vi "OpenLandscape.vi"() -> (1 "Landscape":string[][](array[string]), 2 "Slides":path)   [LabVIEW 2010]
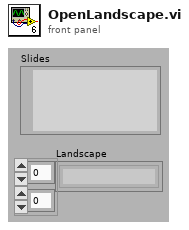
[diagram p1: front panel]
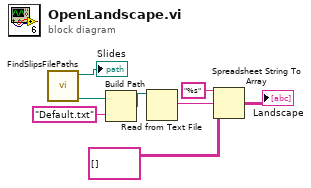
[diagram p0: block diagram]
diagram:
  n1 = call "FindSlipsFilePaths.vi"() -> ("Playlists"=w1:path, "Slides"=→"Slides":path)  [unwired: 2 in, 3 out]
  n2 = Build Path(base path=w1, name or relative path="Default.txt") -> (appended path=w5:path)
  n3 = Read from Text File(file (use dialog)=w5) -> (text=w6:string)  [unwired: 3 in, 3 out]
  n4 = Spreadsheet String To Array(format string="%s", spreadsheet string=w6, array type (2D Dbl)=string[][] [] ("Table Control 2")) -> (array=→"Landscape":string[][])  [unwired: 1 in]
